vi "Test Optionsfeld.vi"() -> ()   [LabVIEW 2015, in "Sprachverwaltung.lvlib"]
uses:
  Sprachverwaltung.lvlib
  Linearisierung V2/AktivButton.ctl
  Linearisierung V2/Linearisierung v2.lvlib
panel:
  in  "Kalibrier Optionen:":enum32{"Gasteiler", "ohne Gasteiler", "PNS"}(radio) caption="Calibration Options:"
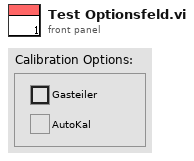
[diagram p1: front panel]
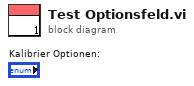
[diagram p0: block diagram]
diagram:
